vi "H(z)toH(w)-DirectIIR.vi"(3 "FFT size":i32=1024, 4 "Reverse":dbl[](array[numeric]), 5 "Forward":dbl[](array[numeric])) -> (0 "df":dbl format="%0.2f", 1 "Phase H(w)":dbl[](array[numeric]) format="%0.2f", 2 "Mag H(w)":dbl[](array[numeric]) format="%0.2f")   [LabVIEW 2021]
uses:
  <vilib>/Analysis/2dsp.llb/Real FFT.vi
  <vilib>/Analysis/NI_AALPro.lvlib
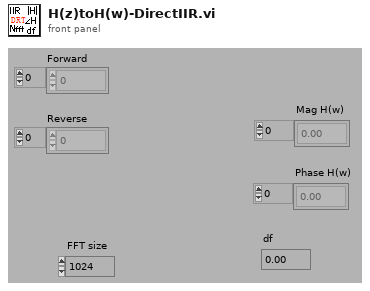
[diagram p1: front panel]
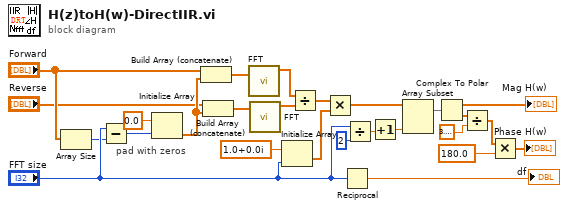
[diagram p0: block diagram]
diagram:
  # "pad with zeros"
  n1 = Array Size(array="Forward") -> (size(s)=w3:i32)
  n2 = Subtract(x="FFT size", y=w3) -> (x-y=w16:i32)
  n3 = Initialize Array(0.0, w16) -> (w15:dbl[])
  n4 = Build Array (concatenate)("Forward", w15) -> (w6:dbl[])
  n5 = Build Array (concatenate)("Reverse", w15) -> (w7:dbl[])
  n6 = call-poly <vilib>:"FFT.vi"("X"=w6) -> ("FFT {X}"=w4:cdb[])  [unwired: 9 in, 1 out]
  n7 = call-poly <vilib>:"FFT.vi"("X"=w7) -> ("FFT {X}"=w5:cdb[])  [unwired: 9 in, 1 out]
  n8 = Initialize Array(cdb 1.0+0.0i, "FFT size") -> (w25:cdb[])
  n9 = Divide(x=w4, y=w5) -> (x/y=w8:cdb[])
  n10 = Multiply(x=w8, y=w25) -> (x*y=w20:cdb[])
  n11 = Reciprocal(x="FFT size") -> (1/x=→"df":dbl)
  n12 = Divide(x="FFT size", y=2) -> (x/y=w23:dbl)
  n13 = Increment(x=w23) -> (x+1=w22:dbl)
  n14 = Array Subset(array=w20, length=w22) -> (w19:cdb[])  [unwired: 1 in]
  n15 = Complex To Polar(r * e^(i*theta)=w19) -> (r=→"Mag H(w)":dbl[], theta=w10:dbl[])
  n16 = Divide(x=w10, y=3.141592653589793) -> (x/y=w11:dbl[])
  n17 = Multiply(x=w11, y=180.0) -> (x*y=→"Phase H(w)":dbl[])
